vi "WPI_PWMChannelCache.vi"(7 "Operation":T2, 8 "error in":errorcluster, 9 "Additional Depth":i32, 11 "PWMChannel":T1=enum."PWM 1") -> (0 "error out":errorcluster, 2 "Allocated?":bool, 3 "AllocatedPWMChannel":T1=enum."PWM 1")   [LabVIEW 2017]
doc: "This software is licensed. Open the labview\\readme\\WPI Robotics Library Open Source License.txt file for more information."
uses:
  <vilib>/Rock Robotics/WPI/PWM/WPI_PWMChannelCacheOp.ctl
  <vilib>/Rock Robotics/SystemInterfaces/DIO/FPGA_DIOPWMChannel.ctl
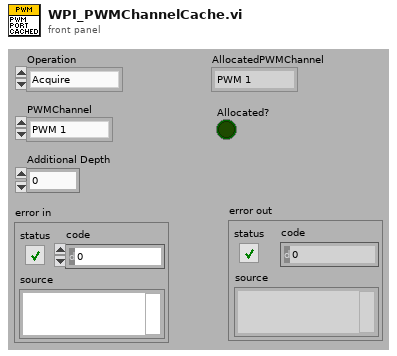
[diagram p1: front panel]
types:
  T1 = typedef "FPGA_DIOPWMChannel.ctl" = enum8{"PWM 0", "PWM 1", "PWM 2", "PWM 3", "PWM 4", "PWM 5", "PWM 6", "PWM 7", "PWM 8", "PWM 9", "PWM MXP 0", "PWM MXP 1", "PWM MXP 2", "PWM MXP 3", "PWM MXP 4", "PWM MXP 5", "PWM MXP 6", "PWM MXP 7", "PWM MXP 8", "PWM MXP 9", "Invalid"}
  T2 = typedef "WPI_PWMChannelCacheOp.ctl" = enum16{"Acquire", "Release", "Status"}
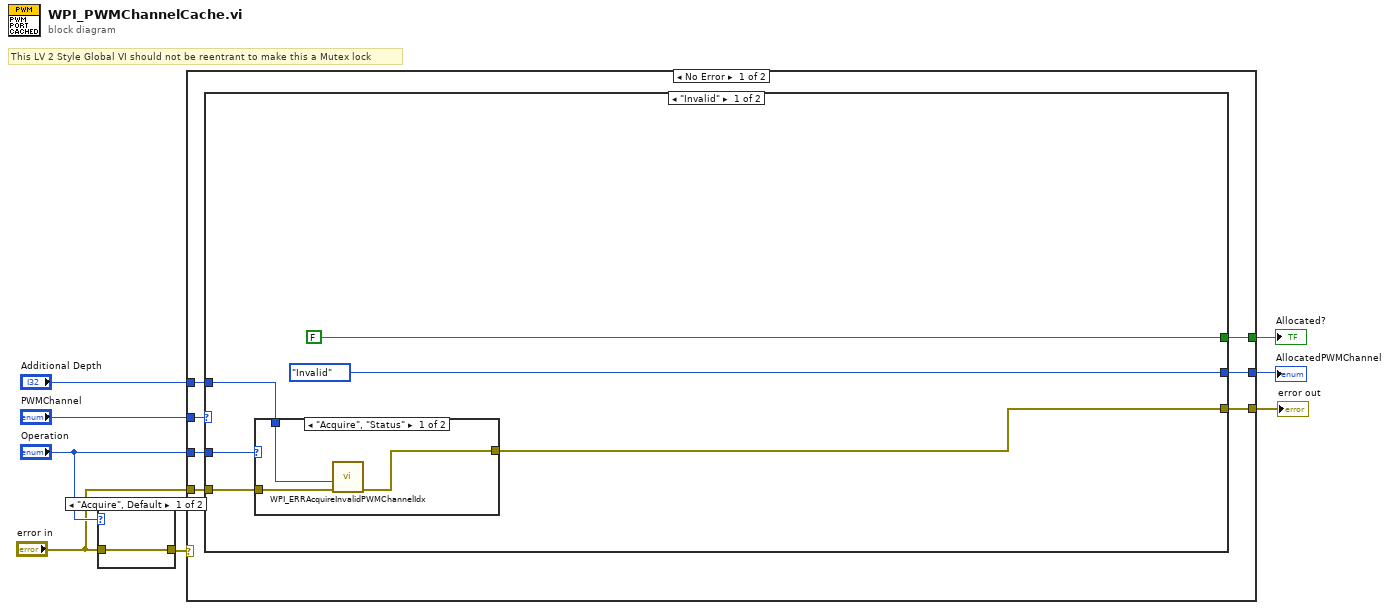
[diagram p0: block diagram]
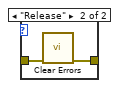
[diagram p2: hidden frame]
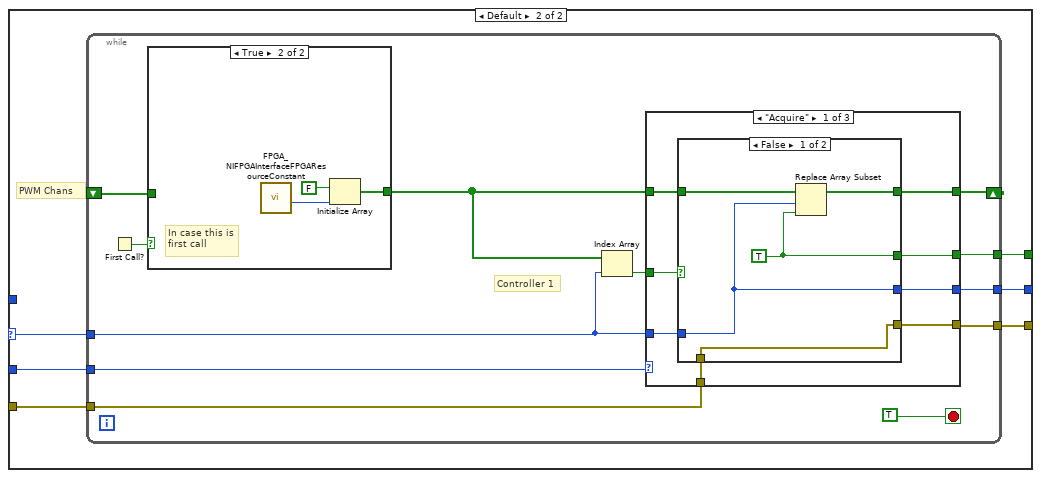
[diagram p4: hidden frame]
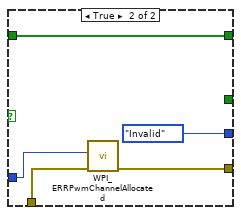
[diagram p5: hidden frame]
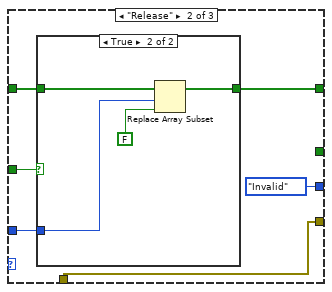
[diagram p6: hidden frame]
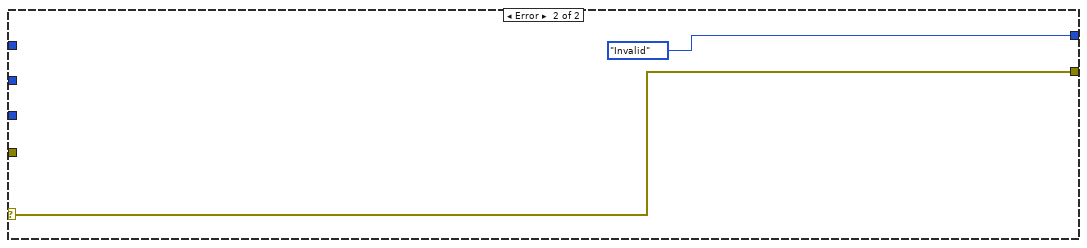
[diagram p10: hidden frame]
diagram:
  # "This LV 2 Style Global VI should not be reentrant to make this a Mutex lock"
  n1 = case shown="\"Acquire\", Default" "Operation" {
    tunnel: "error in" -> [w9 w11]
    tunnel: [w9 w10] -> w7
    frame "Acquire", Default {
    }
    frame "Release" {
      n2 = call <vilib>:"Clear Errors.vi"("error in (no error)"=w11) -> ("error out"=w10:errorcluster)  [unwired: 1 in, 5 out]
    }
  }
  n3 = case shown="No Error" w7 {
    selector: w7 -> [_ w85]
    tunnel: "Operation" -> [w18 _]
    tunnel: "PWMChannel" -> [w17 _]
    tunnel: [w16 w85] -> w3
    tunnel: [w15 _] -> w5
    tunnel: [w14 FPGA_DIOPWMChannel."Invalid" ("AllocatedPWMChannel")] -> w4
    tunnel: "error in" -> [w13 _]
    tunnel: "Additional Depth" -> [w12 _]
    frame No Error {
      n4 = case shown="\"Invalid\"" w17 {
        selector: w17 -> [_ w30]
        tunnel: w18 -> [w24 w34]
        tunnel: [w23 w33] -> w16
        tunnel: [FALSE ("new element/subarray") w32] -> w15
        tunnel: [FPGA_DIOPWMChannel."Invalid" ("AllocatedPWMChannel") w31] -> w14
        tunnel: w13 -> [w20 w29]
        tunnel: w12 -> [w19 _]
        frame "Invalid" {
          n5 = case shown="\"Acquire\", \"Status\"" w24 {
            tunnel: [w27 w28] -> w23
            tunnel: w20 -> [w26 w28]
            tunnel: w19 -> [w25 _]
            frame "Acquire", "Status" {
              n6 = call <vilib>:"WPI_ERRAcquireInvalidPWMChannelIdx.vi"("error in (no error)"=w26, "Additional Depth"=w25) -> ("error in (no error) 2"=w27:errorcluster)  [unwired: 9 in]
            }
            frame "Release" {
            }
          }
        }
        frame Default {
          # "PWM Chans"
          n7 = while {
            shift-right: [w43] -> _
            shift-left: _ -> [w45]
            tunnel: w34 -> [w44]
            tunnel: w30 -> [w39]
            tunnel: [w42] -> w33
            tunnel: [w41] -> w32
            tunnel: [w38] -> w31
            tunnel: w29 -> [w36]
            stop <- TRUE stop-if-true
            # "Controller 1"
            n8 = First Call?() -> (First Call?: T/F=w46:bool)
            n9 = case shown="True" w46 {
              tunnel: w45 -> [w80 _]
              tunnel: [w80 w82] -> w40
              frame False {
              }
              frame True {
                # "In case this is\nfirst call"
                n10 = call <vilib>:"FPGA_NIFPGAInterfaceFPGAResourceConstant.vi"() -> ("NumberOfPWMs"=w81:u32)  [unwired: 11 out]
                n11 = Initialize Array(FALSE, w81) -> (w82:bool[])
              }
            }
            n12 = Index Array(array=w40, index=w39) -> (element=w35:bool)
            n13 = case shown="\"Acquire\"" w44 {
              tunnel: w40 -> [w50 w70 w77]
              tunnel: [w54 w68 w77] -> w43
              tunnel: w39 -> [w53 w69 w79]
              tunnel: [w52 w65 w76] -> w42
              tunnel: [w51 _ w78] -> w41
              tunnel: w35 -> [w49 w67 w78]
              tunnel: [w48 FPGA_DIOPWMChannel."Invalid" ("AllocatedPWMChannel") w79] -> w38
              tunnel: w36 -> [w47 w65 w76]
              frame "Acquire" {
                n14 = case shown="False" w49 {
                  tunnel: w50 -> [w58 w64]
                  tunnel: [w57 w64] -> w54
                  tunnel: w53 -> [w56 w60]
                  tunnel: [w55 w62] -> w52
                  tunnel: [w59 _] -> w51
                  tunnel: [w56 FPGA_DIOPWMChannel."Invalid" ("AllocatedPWMChannel")] -> w48
                  tunnel: w47 -> [w55 w61]
                  frame False {
                    w59 = TRUE ("new element/subarray")
                    n15 = Replace Array Subset(array=w58, new element=w59, index=w56) -> (w57:bool[])
                  }
                  frame True {
                    n16 = call <vilib>:"WPI_ERRPwmChannelAllocated.vi"("error in (no error)"=w61, "PWMChannel"=w60) -> ("ERRPwmChannelAllocated"=w62:errorcluster)  [unwired: 9 in]
                  }
                }
              }
              frame "Release" {
                n17 = case shown="True" w67 {
                  tunnel: w70 -> [w71 w75]
                  tunnel: w69 -> [_ w74]
                  tunnel: [w71 w73] -> w68
                  frame False {
                  }
                  frame True {
                    n18 = Replace Array Subset(array=w75, new element=FALSE ("new element/subarray"), index=w74) -> (w73:bool[])
                  }
                }
              }
              frame "Status" {
              }
            }
          }
        }
      }
    }
    frame Error {
    }
  }
  "Allocated?" <- w5
  "AllocatedPWMChannel" <- w4
  "error out" <- w3
